vi "Map Command Settings.vi"(8 "error in (no error)":errorcluster, 10 "Command Setting Name":string, 11 "Driver in":refnum<class "Driver.lvclass">) -> (0 "error out":errorcluster, 1 "Setting Data Type":string, 2 "Mapped Driver Name":string, 3 "Driver out":refnum<class "Driver.lvclass">)   [LabVIEW 2023, in "HAF.lvlib" / "Driver.lvclass"]
doc: "Converts a mapped Command Setting Name to a Driver Setting Name that is recognisable by the Driver itself. If not recognised by the Driver, \"Ignore\" is returned.\n\nSubclasses must create the mapping structure in order for this to work."
uses:
  Driver.lvclass
  Driver.lvclass/Driver.ctl
  Valid Data Types.ctl
  HAF.lvlib
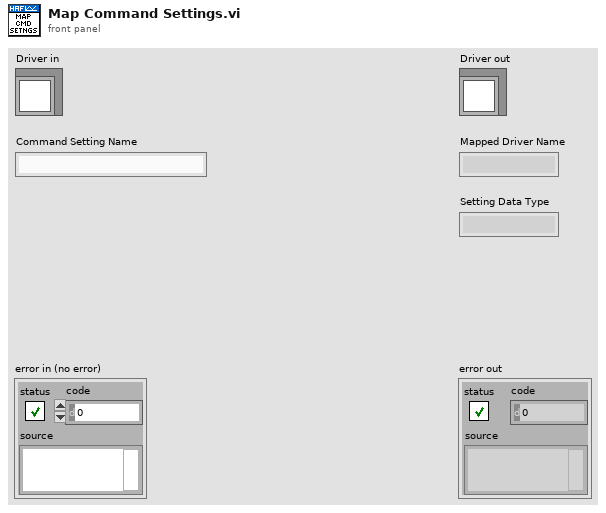
[diagram p1: front panel]
types:
  T1 = typedef "HAF.lvlib/Valid Data Types.ctl" = cluster{"U8":string, "U16":string, "U32":string, "U64":string, "I8":string, "I16 ":string, "I32":string, "I64":string, "SGL":string, "DBL":string, "String":string, "Boolean":string}
  T2 = typedef "HAF.lvlib/Setting Map Structure.ctl" = cluster{"Command Setting Name":string, "Driver Setting Name":string, "Driver Setting Data Type":string}
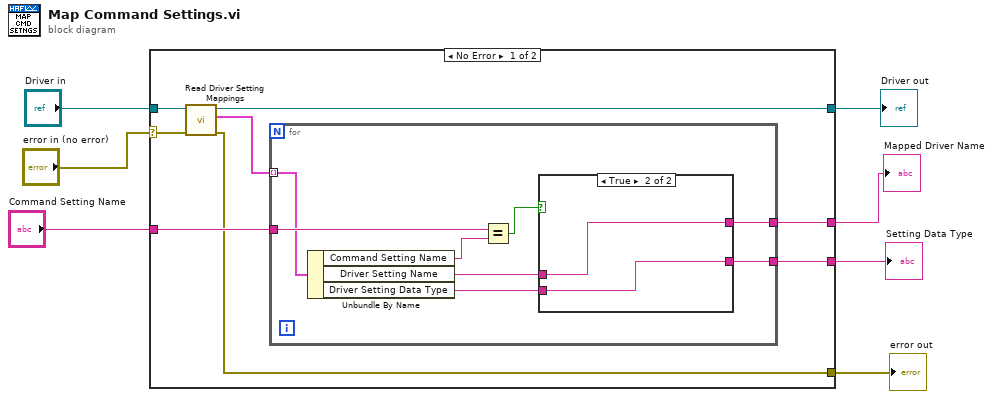
[diagram p0: block diagram]
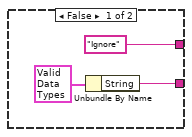
[diagram p2: hidden frame]
diagram:
  n1 = case shown="No Error" "error in (no error)" {
    selector: "error in (no error)" -> [w14 w30]
    tunnel: [w8 w30] -> w6
    tunnel: [w9 w29] -> w4
    tunnel: "Driver in" -> [w15 w29]
    tunnel: "Command Setting Name" -> [w12 _]
    tunnel: [w11 _] -> w2
    tunnel: [w10 _] -> w1
    frame No Error {
      n2 = call-dynamic "Read Driver Setting Mappings.vi"("error in (no error)"=w14, "Driver in"=w15) -> ("error out"=w8:errorcluster, "Driver Setting Mappings"=w13:T2[], "Driver out"=w9:refnum<class "Driver.lvclass">)  [unwired: 7 in]
      n3 = for {
        tunnel: w13 -> [w21] mode=indexing
        tunnel: w12 -> [w23]
        tunnel: [w17] -> w11
        tunnel: [w16] -> w10
        n4 = Unbundle By Name(w21) -> ("Command Setting Name"=w20:string, "Driver Setting Name"=w19:string, "Driver Setting Data Type"=w18:string)
        n5 = Equal?(x=w23, y=w20) -> (x = y?=w22:bool)
        n6 = case shown="True" w22 {
          tunnel: w19 -> [_ w28]
          tunnel: w18 -> [_ w27]
          tunnel: ["Ignore" ("Driver Setting Name") w28] -> w17
          tunnel: [w24 w27] -> w16
          frame False {
            n7 = Unbundle By Name(T1 {"U8"="U8", "U16"="U16", "U32"="U32", "U64"="U64", "I8"="I8", "I16 "="I16", "I32"="I32", "I64"="I64", "SGL"="SGL", "DBL"="DBL", "String"="String", "Boolean"="Boolean"} ("Valid Data Types")) -> ("String"=w24:string)
          }
          frame True {
          }
        }
      }
    }
    frame Error {
    }
  }
  "error out" <- w6
  "Driver out" <- w4
  "Mapped Driver Name" <- w2
  "Setting Data Type" <- w1
